vi "MPErrorMonitor.vi"(0 "Motor DevRefIn":T2={"DeviceStatus"={"status"=FALSE, "code"=0, "source"=""}, "Type"=enum."PWM", "PWM"={"PWM Channel"=enum."PWM 1", "DeadBand"={"Name"="", "maxPositivePwm"=0, "minPositivePwm"=0, "centerPwm"=0, "maxNegativePwm"=0, "minNegativePwm"=0, "angularRange"=0}}, "CAN"={"Device Number"=0, "SetOutput VI Ref"=variant(enum8{"Percent VBus", "Current", "Speed", "Position", "Voltage"} enum."Percent VBus"), "GetOutput VI Ref"=variant(refnum<k1> refnum), "Enable VI Ref"=variant(dbl 12.0), "Disable VI Ref"=variant(enum8{"Percent VBus", "Speed", "Position", "Slave", "Unchanged / Invalid", "Voltage Compensation", "Current", "Motion Profile"} enum."Percent VBus"), "Data"=variant}, "Invert"=FALSE, "DIO PWM"={"PWM \"Enable\" Channel"=enum."Invalid", "DIOChannel"=enum."Invalid", "PWM Rate"=0.0}}, 5 "MotorConfig":T8={"CAN Address"=0, "Invert"=FALSE, "InvertSensor"=FALSE, "Unit Conversion Factor"=0.0, "Brake Mode"=enum."Override to Brake", "Reverse Limt Switch Mode"=enum."Disabled", "Forward Limt Swith Mode"=enum."Disabled", "PWM Channel"=enum."Invalid", "Motor Controller Type"=enum."Talon SRX", "Peak Current (A)"=0, "Continuous Current (A)"=0, "Peak Duration (ms)"=0, "Current Limit Enable"=FALSE}, 7 "Reset":bool, 9 "ErrorThresh (units)":dbl=inf, 11 "error in":errorcluster, 12 "StallDetectTime(ms)":u32=200) -> (3 "Motion Profile Status":T1, 4 "Motor DevRefOut":T2={"DeviceStatus"={"status"=FALSE, "code"=0, "source"=""}, "Type"=enum."PWM", "PWM"={"PWM Channel"=enum."PWM 1", "DeadBand"={"Name"="", "maxPositivePwm"=0, "minPositivePwm"=0, "centerPwm"=0, "maxNegativePwm"=0, "minNegativePwm"=0, "angularRange"=0}}, "CAN"={"Device Number"=0, "SetOutput VI Ref"=variant(enum8{"Percent VBus", "Current", "Speed", "Position", "Voltage"} enum."Percent VBus"), "GetOutput VI Ref"=variant(refnum<k1> refnum), "Enable VI Ref"=variant(dbl 12.0), "Disable VI Ref"=variant(enum8{"Percent VBus", "Speed", "Position", "Slave", "Unchanged / Invalid", "Voltage Compensation", "Current", "Motion Profile"} enum."Percent VBus"), "Data"=variant}, "Invert"=FALSE, "DIO PWM"={"PWM \"Enable\" Channel"=enum."Invalid", "DIOChannel"=enum."Invalid", "PWM Rate"=0.0}}, 6 "Status":T7, 8 "Output Voltage":dbl, 10 "HighError":bool, 13 "Enabled":bool, 14 "Complete":bool, 15 "error out":errorcluster)   [LabVIEW 2018]
uses:
  ArgosLib/Config/ConfigComponents/TypeDefs/Config_Motor.ctl
  <vilib>/Rock Robotics/WPI/ThirdParty/Phoenix-LabVIEW/Motor Controller/Controls/CTRE_Phoenix_MotorControl_NeutralMode.ctl
  <vilib>/Rock Robotics/WPI/ThirdParty/Phoenix-LabVIEW/Motor Controller/Controls/CTRE_Phoenix_MotorControl_LimitSwitchNormal.ctl
  <vilib>/Rock Robotics/SystemInterfaces/DIO/FPGA_DIOPWMChannel.ctl
  ArgosLib/Config/ConfigComponents/TypeDefs/Config_MotorCtrlType.ctl
  <vilib>/Rock Robotics/WPI/MotorControl/WPI_MotorControlDeviceRef.ctl
  <vilib>/Rock Robotics/WPI/MotorControl/WPI_MotorControlType.ctl
  <vilib>/Rock Robotics/WPI/PWM/WPI_PWMDeadband.ctl
  <vilib>/Rock Robotics/SystemInterfaces/DIO/FPGA_DIOChannel.ctl
  <vilib>/Playing With Fusion Inc/Playing With Fusion Lib for FRC/PWF_Venom_LabVIEW/Public/TypeDefs/PwF_Venom_ControlMode.ctl
  <vilib>/Rock Robotics/WPI/ThirdParty/Phoenix-LabVIEW/Motor Controller/Get/CTRE_Phoenix_MotorController_GetVoltage.vi
  <vilib>/Rock Robotics/WPI/ThirdParty/Phoenix-LabVIEW/Motor Controller/Get/CTRE_Phoenix_MotorController_GetSelectedSensorData.vi
  <vilib>/Playing With Fusion Inc/Playing With Fusion Lib for FRC/PWF_Venom_LabVIEW/Public/PwF_Venom_GetControlMode.vi
  <vilib>/Playing With Fusion Inc/Playing With Fusion Lib for FRC/PWF_Venom_LabVIEW/Public/PwF_Venom_GetSpeed.vi
  <vilib>/Playing With Fusion Inc/Playing With Fusion Lib for FRC/PWF_Venom_LabVIEW/Public/PwF_Venom_GetPosition.vi
  <vilib>/Playing With Fusion Inc/Playing With Fusion Lib for FRC/PWF_Venom_LabVIEW/Public/PwF_Venom_GetOutputVoltage.vi
  <vilib>/Playing With Fusion Inc/Playing With Fusion Lib for FRC/PWF_Venom_LabVIEW/PwF_Venom.lvlib
  ArgosLib/ArgosLib.lvlib
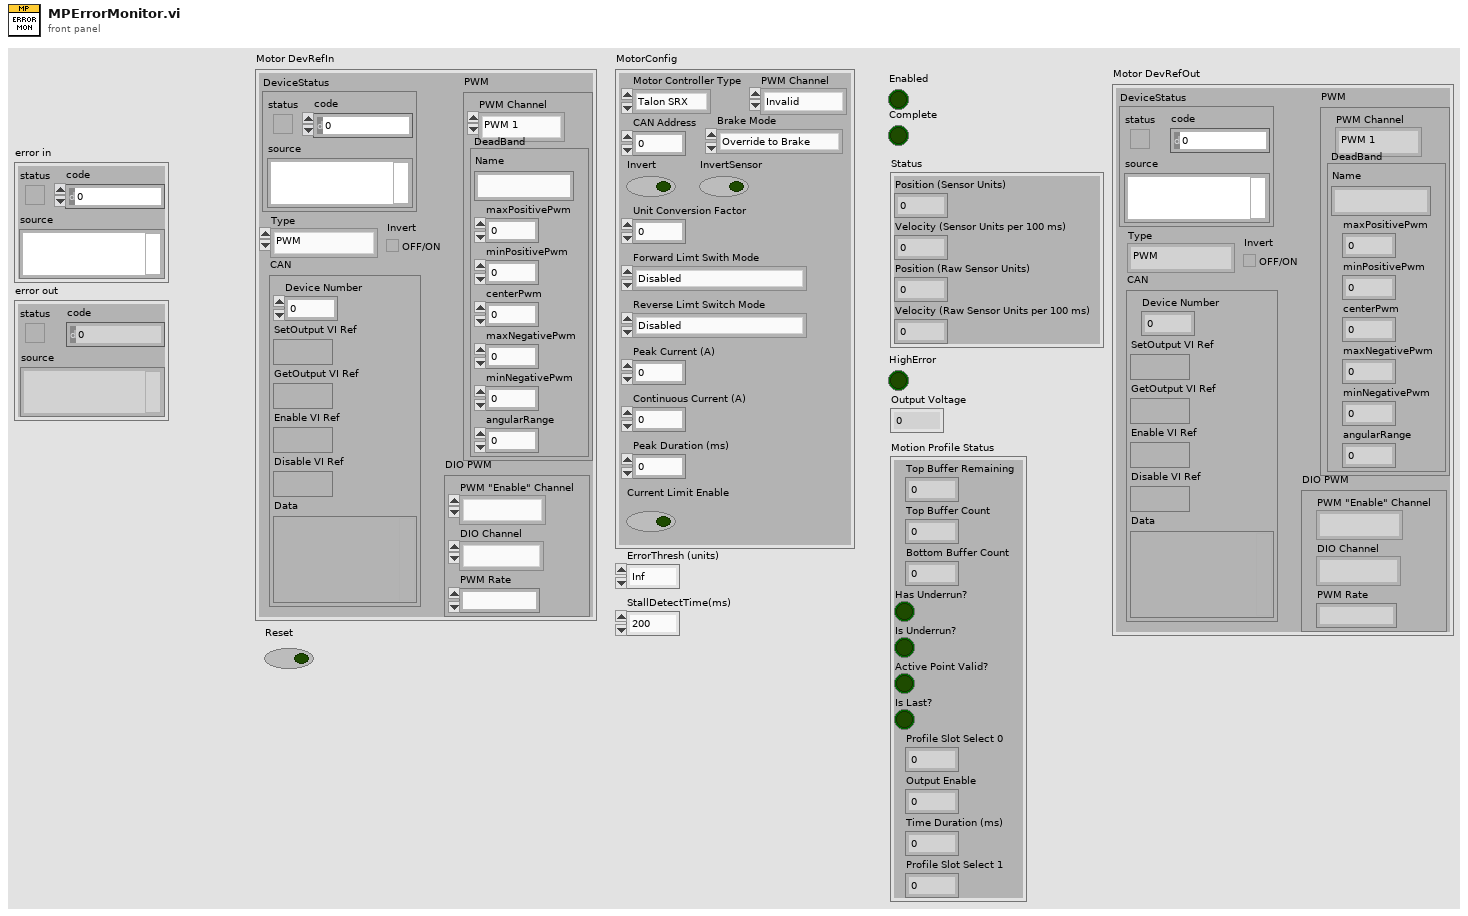
[diagram p1: front panel]
types:
  T1 = cluster{"Top Buffer Remaining":i32, "Top Buffer Count":i32, "Bottom Buffer Count":i32, "Has Underrun?":bool, "Is Underrun?":bool, "Active Point Valid?":bool, "Is Last?":bool, "Profile Slot Select 0":i32, "Output Enable":i32, "Time Duration (ms)":i32, "Profile Slot Select 1":i32}
  T2 = typedef "WPI_MotorControlDeviceRef.ctl" = cluster{"DeviceStatus":errorcluster, "Type":T3, "PWM":cluster{"PWM Channel":T4, "DeadBand":T5}, "CAN":cluster{"Device Number":u8, "SetOutput VI Ref":variant, "GetOutput VI Ref":variant, "Enable VI Ref":variant, "Disable VI Ref":variant, "Data":variant}, "Invert":bool, "DIO PWM":cluster{"PWM \"Enable\" Channel":T4, "DIOChannel":T6, "PWM Rate":dbl}}
  T3 = typedef "WPI_MotorControlType.ctl" = enum16{"PWM", "CAN", "DIO PWM"}
  T4 = typedef "FPGA_DIOPWMChannel.ctl" = enum8{"PWM 0", "PWM 1", "PWM 2", "PWM 3", "PWM 4", "PWM 5", "PWM 6", "PWM 7", "PWM 8", "PWM 9", "PWM MXP 0", "PWM MXP 1", "PWM MXP 2", "PWM MXP 3", "PWM MXP 4", "PWM MXP 5", "PWM MXP 6", "PWM MXP 7", "PWM MXP 8", "PWM MXP 9", "Invalid"}
  T5 = typedef "WPI_PWMDeadband.ctl" = cluster{"Name":string, "maxPositivePwm":i32, "minPositivePwm":i32, "centerPwm":i32, "maxNegativePwm":i32, "minNegativePwm":i32, "angularRange":u16}
  T6 = typedef "FPGA_DIOChannel.ctl" = enum8{"DIO 0", "DIO 1", "DIO 2", "DIO 3", "DIO 4", "DIO 5", "DIO 6", "DIO 7", "DIO 8", "DIO 9", "DIO MXP 0", "DIO MXP 1", "DIO MXP 2", "DIO MXP 3", "DIO MXP 4", "DIO MXP 5", "DIO MXP 6", "DIO MXP 7", "DIO MXP 8", "DIO MXP 9", "DIO MXP 10", "DIO MXP 11", "DIO MXP 12", "DIO MXP 13", "DIO MXP 14", "DIO MXP 15", "SPI Port CS1", "SPI Port CS2", "SPI Port CS3", "SPI Port MISO", "SPI Port MOSI", "Invalid"}
  T7 = cluster{"Position (Sensor Units)":dbl, "Velocity (Sensor Units per 100 ms)":dbl, "Position (Raw Sensor Units)":dbl, "Velocity (Raw Sensor Units per 100 ms)":dbl}
  T8 = typedef "ArgosLib.lvlib/Config_Motor.ctl" = cluster{"CAN Address":u8, "Invert":bool, "InvertSensor":bool, "Unit Conversion Factor":dbl, "Brake Mode":T9, "Reverse Limt Switch Mode":T10, "Forward Limt Swith Mode":T10, "PWM Channel":T4, "Motor Controller Type":T11, "Peak Current (A)":i32, "Continuous Current (A)":i32, "Peak Duration (ms)":i32, "Current Limit Enable":bool}
  T9 = typedef "CTRE_Phoenix_MotorControl_NeutralMode.ctl" = enum8{"EEPROMSetting", "Override to Coast", "Override to Brake"}
  T10 = typedef "CTRE_Phoenix_MotorControl_LimitSwitchNormal.ctl" = enum16{"Normally Open", "Normally Closed", "Disabled"}
  T11 = typedef "ArgosLib.lvlib/Config_MotorCtrlType.ctl" = enum16{"Disabled", "Talon SRX", "Talon SR", "Venom"}
  T12 = cluster{"Position":dbl, "Speed":dbl, "TargetPosition":dbl, "TargetPosition":dbl}
  T13 = cluster{"Position (Sensor Units)":i32, "Velocity (Sensor Units per 100 ms)":i32, "Position (Raw Sensor Units)":i32, i32}
  T14 = typedef "PlayingWithFusionLib.lvlib/PwF_Venom.lvlib/PwF_Venom_ControlMode.ctl" = u8
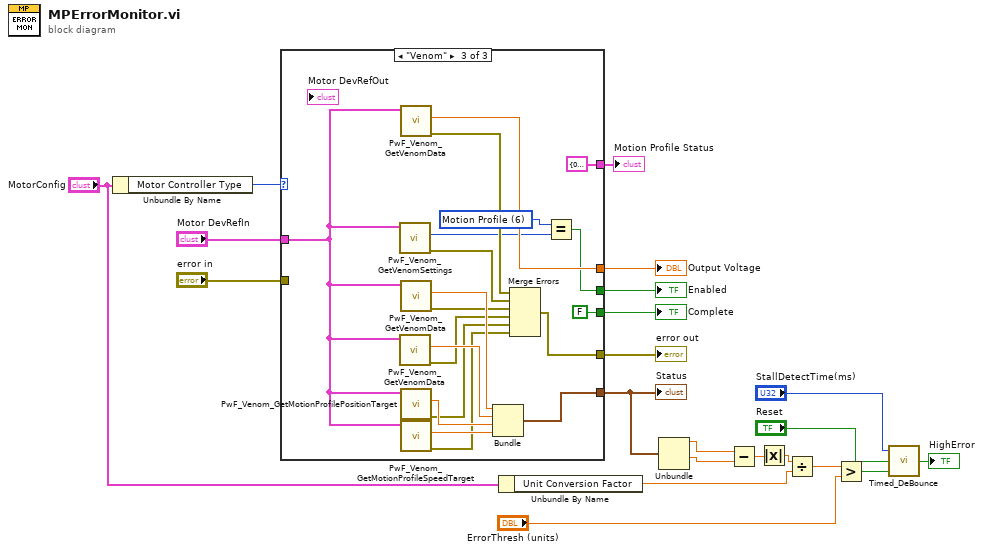
[diagram p0: block diagram]
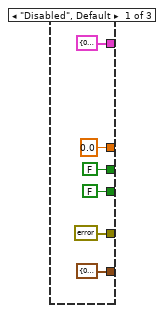
[diagram p2: hidden frame]
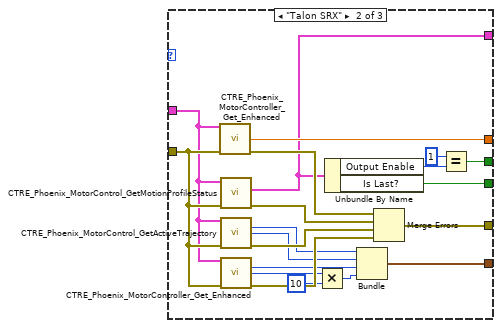
[diagram p3: hidden frame]
diagram:
  n1 = Unbundle By Name("MotorConfig") -> ("Motor Controller Type"=w18:T11)
  n2 = case shown="\"Venom\"" w18 {
    tunnel: [errorcluster {"status"=FALSE, "code"=0, "source"=""} ("error IO") w43 w54] -> w21
    tunnel: "error in" -> [_ w42 _]
    tunnel: "Motor DevRefIn" -> [_ w41 w52]
    tunnel: [T12 {"Position"=0.0, "Speed"=0.0, "TargetPosition"=0.0, "TargetPosition"=0.0} w34 w61] -> w8
    tunnel: [0.0 ("Output Voltage") w33 w66] -> w17
    tunnel: [FALSE w30 w48] -> w16
    tunnel: [FALSE ("Is Last?") w29 FALSE ("Is Last?")] -> w15
    tunnel: [T1 {"Top Buffer Remaining"=0, "Top Buffer Count"=0, "Bottom Buffer Count"=0, "Has Underrun?"=FALSE, "Is Underrun?"=FALSE, "Active Point Valid?"=FALSE, "Is Last?"=FALSE, "Profile Slot Select 0"=0, "Output Enable"=0, "Time Duration (ms)"=0, "Profile Slot Select 1"=0} ("Motion Profile Status") w28 T1 {"Top Buffer Remaining"=0, "Top Buffer Count"=0, "Bottom Buffer Count"=0, "Has Underrun?"=FALSE, "Is Underrun?"=FALSE, "Active Point Valid?"=FALSE, "Is Last?"=FALSE, "Profile Slot Select 0"=0, "Output Enable"=0, "Time Duration (ms)"=0, "Profile Slot Select 1"=0} ("Motion Profile Status")] -> w1
    frame "Disabled", Default {
    }
    frame "Talon SRX" {
      n3 = call-poly <vilib>:"CTRE_Phoenix_MotorController_Get_Enhanced.vi"("PhoenixMotorControlDevRef"=w41, "error in"=w42) -> ("Output Voltage"=w33:dbl, "error out"=w44:errorcluster)  [unwired: 9 in, 3 out]
      n4 = call <vilib>:"CTRE_Phoenix_MotorControl_GetMotionProfileStatus.vi"("error in"=w42, "PhoenixMotorControlDevRef"=w41) -> ("error out"=w47:errorcluster, "Motion Profile Status"=w28:T1)  [unwired: 7 in, 1 out]
      n5 = call <vilib>:"CTRE_Phoenix_MotorControl_GetActiveTrajectory.vi"("PhoenixMotorControlDevRef"=w41, "error in"=w42) -> ("Position (Sensor Units)"=w40:i32, "Velocity (Sensor Units per 100 ms)"=w39:i32, "error out"=w46:errorcluster)  [unwired: 9 in, 2 out]
      n6 = call-poly <vilib>:"CTRE_Phoenix_MotorController_Get_Enhanced.vi"("PhoenixMotorControlDevRef"=w41, "error in"=w42) -> ("Position (Raw Sensor Units)"=w38:i32, "Velocity (Raw Sensor Units per 100 ms)"=w36:i32, "error out"=w45:errorcluster)  [unwired: 10 in, 1 out]
      n7 = Multiply(x=w36, y=10) -> (x*y=w37:i32)
      n8 = Unbundle By Name(w28) -> ("Output Enable"=w32:i32, "Is Last?"=w29:bool)
      n9 = Bundle("Position (Sensor Units)"=w40, "Velocity (Sensor Units per 100 ms)"=w39, "Position (Raw Sensor Units)"=w38, w37) -> (w34:T13)  [unwired: 1 in]
      n10 = Merge Errors(w44, w47, w46, w45) -> (w43:errorcluster)
      n11 = Equal?(x=1, y=w32) -> (x = y?=w30:bool)
    }
    frame "Venom" {
      w49 = T14 6 items=["Disabled"=0, "Proportional"=1, "Current Control"=3, "Speed Control"=4, "Position Control"=5, "Motion Profile"=6, "Follow The Leader"=7, "Voltage Control"=8] ("x")
      n12 = call-poly <vilib>:"PwF_Venom_GetVenomSettings.vi"("PwFVenomDevRefIn"=w52) -> ("error out"=w51:errorcluster, "PwF Venom Control Mode"=w50:T14)  [unwired: 8 in, 1 out]
      n13 = call-poly <vilib>:"PwF_Venom_GetVenomData.vi"("PwFVenomDevRefIn"=w52) -> ("error out"=w57:errorcluster, "Speed"=w64:dbl)  [unwired: 8 in, 1 out]
      n14 = call-poly <vilib>:"PwF_Venom_GetVenomData.vi"("PwFVenomDevRefIn"=w52) -> ("error out"=w59:errorcluster, "Output Voltage"=w66:dbl)  [unwired: 8 in, 1 out]
      n15 = call-poly <vilib>:"PwF_Venom_GetVenomData.vi"("PwFVenomDevRefIn"=w52) -> ("error out"=w58:errorcluster, "Position"=w65:dbl)  [unwired: 8 in, 1 out]
      n16 = call <vilib>:"PwF_Venom_GetMotionProfilePositionTarget.vi"("PwFVenomDevRefIn"=w52) -> ("error out"=w56:errorcluster, "TargetPosition"=w63:dbl)  [unwired: 8 in, 1 out]
      n17 = call <vilib>:"PwF_Venom_GetMotionProfileSpeedTarget.vi"("PwFVenomDevRefIn"=w52) -> ("error out"=w55:errorcluster, "TargetPosition"=w62:dbl)  [unwired: 8 in, 1 out]
      n18 = Bundle("Position"=w65, "Speed"=w64, "TargetPosition"=w63, "TargetPosition"=w62) -> (w61:T12)  [unwired: 1 in]
      n19 = Merge Errors(w59, w51, w58, w57, w56, w55) -> (w54:errorcluster)
      n20 = Equal?(x=w49, y=w50) -> (x = y?=w48:bool)
    }
  }
  "Enabled" <- w16
  "Complete" <- w15
  "Status" <- w8
  "error out" <- w21
  "Output Voltage" <- w17
  "Motion Profile Status" <- w1
  n21 = Unbundle By Name("MotorConfig") -> ("Unit Conversion Factor"=w6:dbl)
  n22 = Unbundle(w8) -> ("Position"=w11:dbl, "TargetPosition"=w10:dbl)  [unwired: 2 out]
  n23 = Subtract(x=w11, y=w10) -> (x-y=w12:dbl)
  n24 = Absolute Value(x=w12) -> (abs(x)=w9:dbl)
  n25 = Divide(x=w9, y=w6) -> (x/y=w14:dbl)
  n26 = Greater?(x=w14, y="ErrorThresh (units)") -> (0:w13:bool)
  n27 = call "Timed_DeBounce.vi"("Input"=w13, "Reset"="Reset", "Hold Time(ms)"="StallDetectTime(ms)") -> ("Output"=→"HighError":bool)
